vi "MatchingDiceMarcoGonzalez.vi"() -> ()   [LabVIEW 2012]
doc: "This VI will roll 2 die and will stop when both die match. It will keep track of how many times it took to match the die."
panel:
  out "Number on Dice 2":dbl
  out "Number on Dice 1":dbl
  out "Rolls":dbl
  # "Marco Gonzalez\nEA 3\n03 / 03 /2017"
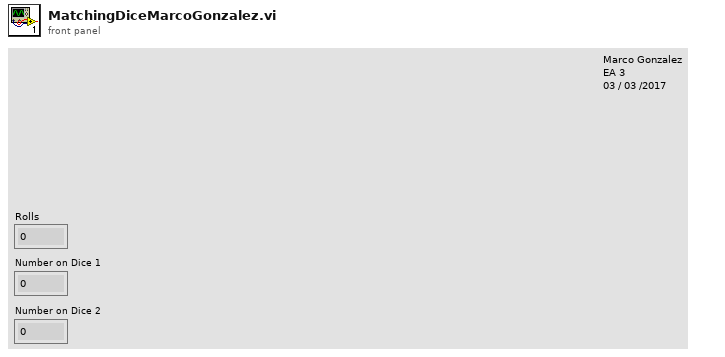
[diagram p1: front panel]
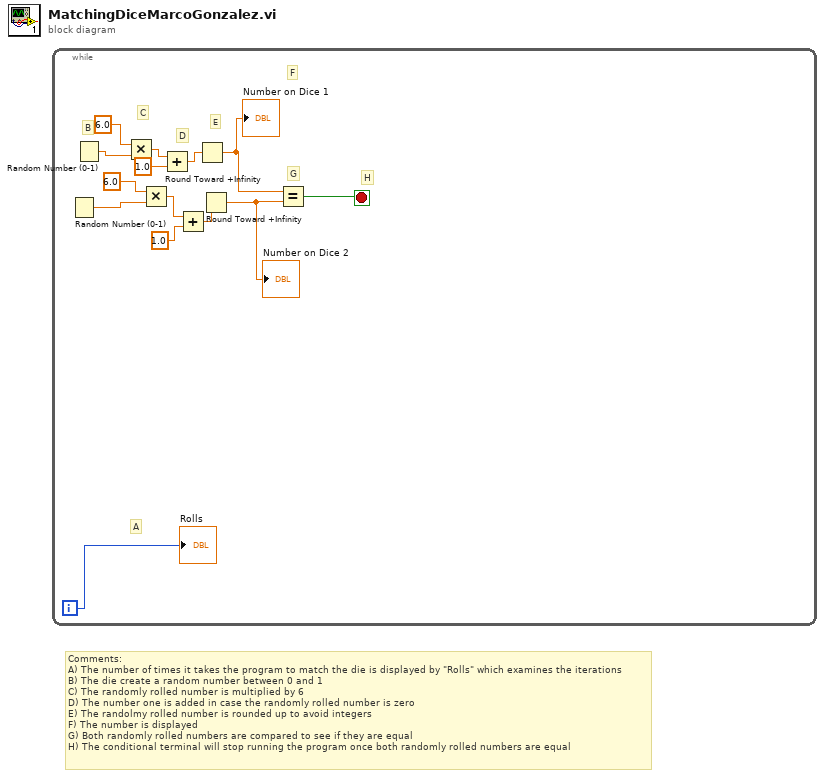
[diagram p0: block diagram]
diagram:
  # "Comments:\nA) The number of times it takes the program to match the die is displayed by \"Rolls\" which examines the iterations\nB) The die create a random number between 0 and 1\nC) The randomly rolled number is multiplied by 6\nD) The number one is added in case the randomly rolled number is zero\nE) The randolmy rolled number is rounded up to avoid integers\nF) The number is displayed\nG) Both randomly rolled numbers are compared to see if they are equal\nH) The conditional terminal will stop running the program once both randomly rolled numbers are equal"
  n1 = while {
    i -> [w14]
    stop <- w13 stop-if-true
    # "H"
    # "G"
    # "F"
    # "E"
    # "D"
    # "C"
    # "B"
    # "A"
    n2 = Random Number (0-1)() -> (number: 0 to 1=w5:dbl)
    n3 = Random Number (0-1)() -> (number: 0 to 1=w11:dbl)
    n4 = Multiply(x=6.0, y=w11) -> (x*y=w9:dbl)
    n5 = Multiply(x=6.0, y=w5) -> (x*y=w3:dbl)
    n6 = Add(x=w9, y=1.0) -> (x+y=w7:dbl)
    n7 = Add(x=w3, y=1.0) -> (x+y=w1:dbl)
    n8 = Round Toward +Infinity(x=w7) -> (ceil(x): smallest int >= x=w12:dbl)
    "Number on Dice 1" <- w12
    n9 = Round Toward +Infinity(x=w1) -> (ceil(x): smallest int >= x=w6:dbl)
    "Number on Dice 2" <- w6
    n10 = Equal?(x=w12, y=w6) -> (x = y?=w13:bool)
    "Rolls" <- w14
  }
